vi "niScope Cleanup Digitizing Process.vi"(8 "error in":errorcluster, 11 "niScope in":T1={"channel cfg"=[], "sessions"=[], "multi cards"=FALSE, "channels"=0, "type"=enum."n/a", "memory [B/chn]"=0, "ext. clock [Hz]"=0.0, "samples count"=0, "use streaming"=FALSE, "proc setup"={"packet size [smpl]"=0, "current timeout [s]"=0.0, "blk2blk timeout [s]"=0.0, "event time"=timestamp(0 s since 1904-01-01), "temp sampl T [s]"=0.0, "data queue"=refnum, "stop notifier"=refnum, "proc ref"=refnum}, "sample width [B]"=0, "ranges [V]"=[], "trigger setup"={"coupling"=1, "level [V]"=0.0, "slope"=0, "mode"=enum."Immediate"}, "fs [Hz]"=0.0, "bitres [bit]"=0} {"trigger setup"."level [V]" format="%.2f"; "trigger setup"."coupling" items=["AC"=0, "DC"=1, "HF Reject"=3, "LF Reject"=4, "AC Plus HF Reject"=1001]; "channel cfg"."Range [Vpk]" min=0.0; "channel cfg"."Channel" min=0}) -> (0 "error out":errorcluster, 3 "niScope out":T1={"channel cfg"=[], "sessions"=[], "multi cards"=FALSE, "channels"=0, "type"=enum."n/a", "memory [B/chn]"=0, "ext. clock [Hz]"=0.0, "samples count"=0, "use streaming"=FALSE, "proc setup"={"packet size [smpl]"=0, "current timeout [s]"=0.0, "blk2blk timeout [s]"=0.0, "event time"=timestamp(0 s since 1904-01-01), "temp sampl T [s]"=0.0, "data queue"=refnum, "stop notifier"=refnum, "proc ref"=refnum}, "sample width [B]"=0, "ranges [V]"=[], "trigger setup"={"coupling"=1, "level [V]"=0.0, "slope"=0, "mode"=enum."Immediate"}, "fs [Hz]"=0.0, "bitres [bit]"=0} {"trigger setup"."level [V]" format="%.2f"; "trigger setup"."coupling" items=["AC"=0, "DC"=1, "HF Reject"=3, "LF Reject"=4, "AC Plus HF Reject"=1001]; "channel cfg"."Range [Vpk]" min=0.0; "channel cfg"."Channel" min=0})   [LabVIEW 2018, in "niScope Virtual Digitizer.lvlib"]
doc: "Cleans up everything related to the digitizing process. Must be called after each use of Initiate Digitizing Process to deallocate all related objects and to stop Digitizing Process. It must be called even if digitizing failed or was aborted!\nThe VI ignores input error so it will always execute."
uses:
  niScope Virtual Digitizer.lvlib
  niScope Session.ctl
  niScope Virtual Channel Config.ctl
  niScope Virtual Channel Mode.ctl
  niScope Virtual Channel Input Z.ctl
  niScope Virtual Channel Coupling.ctl
  niScope Type.ctl
  niScope Digitizing Process Options.ctl
  niScope Data Packet.ctl
  niScope Trigger Setup.ctl
  <instrlib>/niScope/Controls/niScope trigger coupling.ctl
  <instrlib>/niScope/Controls/niScope trigger slope.ctl
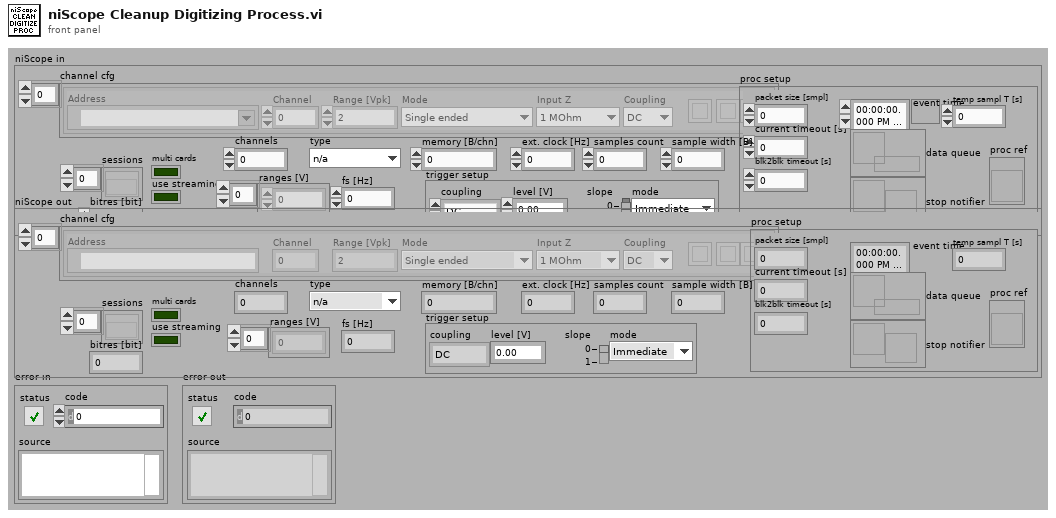
[diagram p1: front panel]
types:
  T1 = typedef "niScope Virtual Digitizer.lvlib/niScope Session.ctl" = cluster{"channel cfg":T2[], "sessions":refnum<k20>[], "multi cards":bool, "channels":i32, "type":T6, "memory [B/chn]":i32, "ext. clock [Hz]":dbl, "samples count":i64, "use streaming":bool, "proc setup":T7, "sample width [B]":i32, "ranges [V]":dbl[], "trigger setup":T8, "fs [Hz]":dbl, "bitres [bit]":i32}
  T2 = typedef "niScope Virtual Digitizer.lvlib/niScope Virtual Channel Config.ctl" = cluster{"Address":refnum<k15>, "Channel":i32, "Mode":T3, "Input Z":T4, "Coupling":T5, "Range [Vpk]":dbl, "btn clr":bool, "btn up":bool, "btn down":bool}
  T3 = typedef "niScope Virtual Digitizer.lvlib/niScope Virtual Channel Mode.ctl" = enum16{"Single ended", "Unbal. differential", "Differential"}
  T4 = typedef "niScope Virtual Digitizer.lvlib/niScope Virtual Channel Input Z.ctl" = enum16{"1 MOhm", "50 Ohm"}
  T5 = typedef "niScope Virtual Digitizer.lvlib/niScope Virtual Channel Coupling.ctl" = enum16{"AC", "DC", "GND"}
  T6 = typedef "niScope Virtual Digitizer.lvlib/niScope Type.ctl" = enum16{"n/a", "5922"}
  T7 = typedef "niScope Virtual Digitizer.lvlib/niScope Digitizing Process Options.ctl" = cluster{"packet size [smpl]":i64, "current timeout [s]":dbl, "blk2blk timeout [s]":dbl, "event time":timestamp, "temp sampl T [s]":dbl, "data queue":refnum<queue>, "stop notifier":refnum<notifier>, "proc ref":refnum<vi>}
  T8 = typedef "niScope Virtual Digitizer.lvlib/niScope Trigger Setup.ctl" = cluster{"coupling":T9, "level [V]":dbl, "slope":T10, "mode":enum16{"Immediate", "External", "Level"}}
  T9 = typedef "niScope trigger coupling.ctl" = u16
  T10 = typedef "niScope trigger slope.ctl" = i32
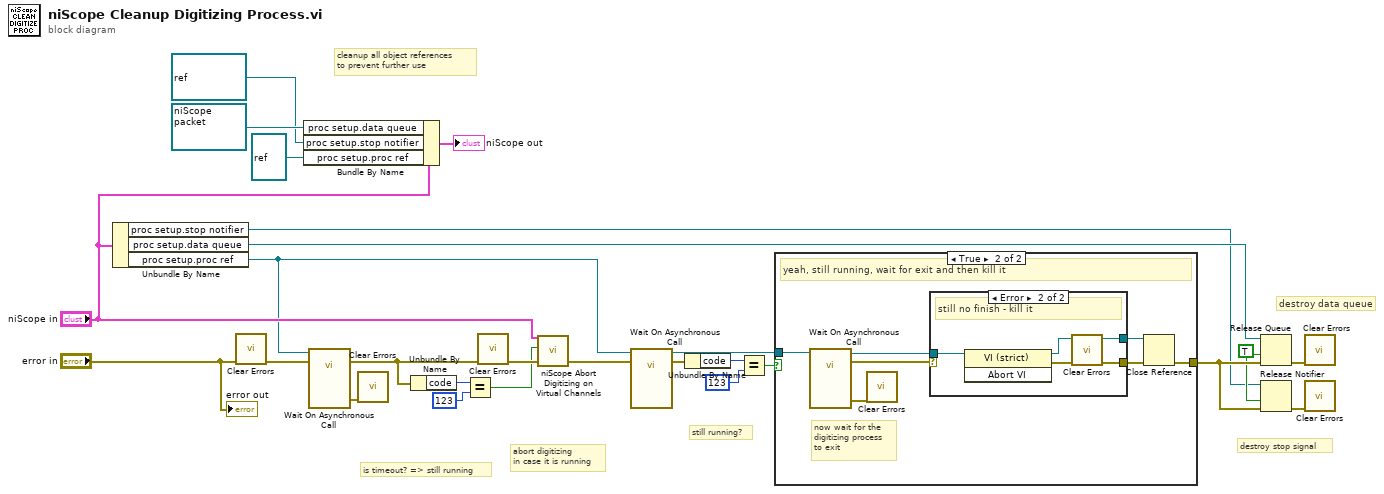
[diagram p0: block diagram]
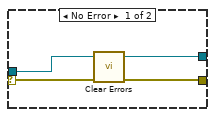
[diagram p3: hidden frame]
diagram:
  w21 = TRUE ("force destroy? (F)")
  # "still running?"
  # "abort digitizing\nin case it is running"
  # "cleanup all object references\nto prevent further use"
  # "destroy stop signal"
  # "destroy data queue"
  # "is timeout? => still running"
  n1 = Unbundle By Name("niScope in") -> ("proc setup.stop notifier"=w20:refnum<notifier>, "proc setup.data queue"=w23:refnum<queue>, "proc setup.proc ref"=w6:refnum<vi>)
  n2 = call <vilib>:"Clear Errors.vi"("error in (no error)"="error in") -> ("error out"=w13:errorcluster)  [unwired: 5 in, 1 out]
  n3 = Bundle By Name(cluster="niScope in", "proc setup.data queue"=refnum<queue> refnum, "proc setup.stop notifier"=refnum<notifier> refnum, "proc setup.proc ref"=refnum<vi> refnum) -> (→"niScope out":T1)
  n4 = call-by-ref "Wait On Asynchronous Call"(reference=w6, error in=w13) -> (error out=w11:errorcluster, 0:"error out"=w12:errorcluster)  [unwired: 10 in, 2 out]
  n5 = call <vilib>:"Clear Errors.vi"("error in (no error)"=w12) -> ()  [unwired: 5 in, 2 out]
  n6 = Unbundle By Name(w11) -> ("code"=w10:i32)
  n7 = Equal?(x=w10, y=123) -> (x = y?=w8:bool)
  n8 = call <vilib>:"Clear Errors.vi"("error in (no error)"=w11) -> ("error out"=w26:errorcluster)  [unwired: 5 in, 1 out]
  n9 = call "niScope Abort Digitizing on Virtual Channels.vi"("error in"=w26, "abort (True)"=w8, "niScope in"="niScope in") -> ("error out"=w7:errorcluster)  [unwired: 7 in, 1 out]
  n10 = call-by-ref "Wait On Asynchronous Call"(reference=w6, error in=w7) -> (reference out=w1:refnum<vi>, error out=w5:errorcluster)  [unwired: 10 in, 2 out]
  n11 = Unbundle By Name(w5) -> ("code"=w4:i32)
  n12 = Equal?(x=w4, y=123) -> (x = y?=w2:bool)
  n13 = case shown="True" w2 {
    tunnel: [_ w28] -> w22
    tunnel: w1 -> [_ w30]
    frame False {
    }
    frame True {
      # "now wait for the\ndigitizing process\nto exit"
      # "yeah, still running, wait for exit and then kill it"
      n14 = call-by-ref "Wait On Asynchronous Call"(reference=w30) -> (reference out=w32:refnum<vi>, error out=w33:errorcluster, 0:"error out"=w31:errorcluster)  [unwired: 11 in, 1 out]
      n15 = call <vilib>:"Clear Errors.vi"("error in (no error)"=w31) -> ()  [unwired: 5 in, 2 out]
      n16 = case shown="Error" w33 {
        selector: w33 -> [w35 _]
        tunnel: w32 -> [w34 w40]
        tunnel: [w36 w38] -> w29
        tunnel: [w34 w37] -> w27
        frame No Error {
          n17 = call <vilib>:"Clear Errors.vi"("error in (no error)"=w35) -> ("error out"=w36:errorcluster)  [unwired: 5 in, 1 out]
        }
        frame Error {
          # "still no finish - kill it"
          n18 = invoke class="VI (strict)" method="Abort VI"(reference=w40) -> (reference out=w37:refnum<vi>, error out=w39:errorcluster)  [unwired: 2 in, 1 out]
          n19 = call <vilib>:"Clear Errors.vi"("error in (no error)"=w39) -> ("error out"=w38:errorcluster)  [unwired: 5 in, 1 out]
        }
      }
      n20 = Close Reference(reference=w27, error in (no error)=w29) -> (error out=w28:errorcluster)
    }
  }
  n21 = Release Queue(queue=w23, force destroy? (F)=w21, error in (no error)=w22) -> (error out=w25:errorcluster)  [unwired: 2 out]
  n22 = Release Notifier(notifier=w20, force destroy? (F)=w21, error in (no error)=w22) -> (error out=w14:errorcluster)  [unwired: 2 out]
  n23 = call <vilib>:"Clear Errors.vi"("error in (no error)"=w25) -> ()  [unwired: 5 in, 2 out]
  n24 = call <vilib>:"Clear Errors.vi"("error in (no error)"=w14) -> ()  [unwired: 5 in, 2 out]
  "error out" <- "error in"
